vi "NIRFSG_SetBW.vi"(8 "error in (no error)":errorcluster, 10 "Addr./Alias":string, 11 "Controls":variant) -> (0 "error out":errorcluster, 3 "Results":variant)   [LabVIEW 2015]
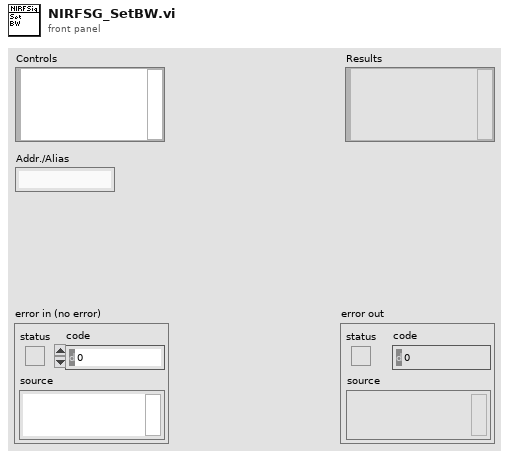
[diagram p1: front panel]
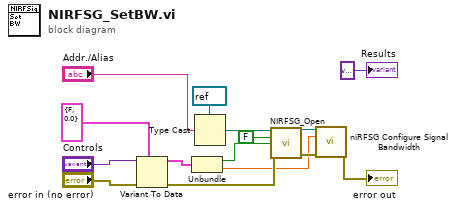
[diagram p0: block diagram]
diagram:
  n1 = Variant To Data(error in="error in (no error)", type=cluster{"Open Session":bool, "BW (Hz)":dbl} {"Open Session"=FALSE, "BW (Hz)"=0.0}, Variant="Controls") -> (data=w4:cluster{"Open Session":bool, "BW (Hz)":dbl}, error out=w10:errorcluster)
  n2 = Unbundle(w4) -> ("Open Session"=w2:bool, "BW (Hz)"=w1:dbl)
  n3 = Type Cast(type=refnum<k15> refnum ("instrument handle"), x="Addr./Alias") -> (*(type *) &x=w11:refnum<k15>)
  n4 = call "NIRFSG_Open.vi"("Session Name"=w11, "Reset Instr"=FALSE, "Open Session"=w2, "error in (no error)"=w10) -> ("instrument handle out"=w8:refnum<k15>, "error out"=w7:errorcluster)  [unwired: 10 in]
  n5 = call <instrlib>:"niRFSG Configure Signal Bandwidth.vi"("instrument handle"=w8, "signal bandwidth (Hz)"=w1, "error in"=w7) -> ("error out"=→"error out":errorcluster)  [unwired: 11 in, 1 out]
  "Results" <- variant ("Results")
